vi "加载compactRIOconfig.vi"(8 "error in (no error)":errorcluster caption="错误输入（无错误）") -> (0 "error out":errorcluster caption="错误输出")   [LabVIEW 2014]
doc: "该模板用于创建子VI。"
uses:
  glb/glb_static.vi
  <vilib>/Utility/config.llb/NI_LVConfig.lvlib
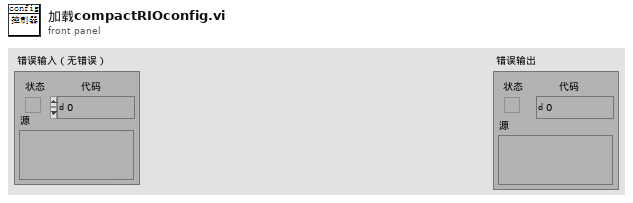
[diagram p1: front panel]
types:
  T1 = typedef "NI_LVConfig.lvlib/Config Data RefNum.ctl" = refnum<k1>
  T2 = cluster{"板卡类型":string, "信号类型":string, "上限":string, "下限":string, "单位":string, "通道数":u32, "最大采样率":u32, "设置采样率":u32, "附加条件":string[], "板卡型号":string}
  T3 = cluster{"控制型号":string, "插槽数目":u32, "板卡信息":cluster{"板卡类型":string, "信号类型":string, "上限":string, "下限":string, "单位":string, "通道数":u32, "最大采样率":u32, "设置采样率":u32, "附加条件":string[], "板卡型号":string}[]}
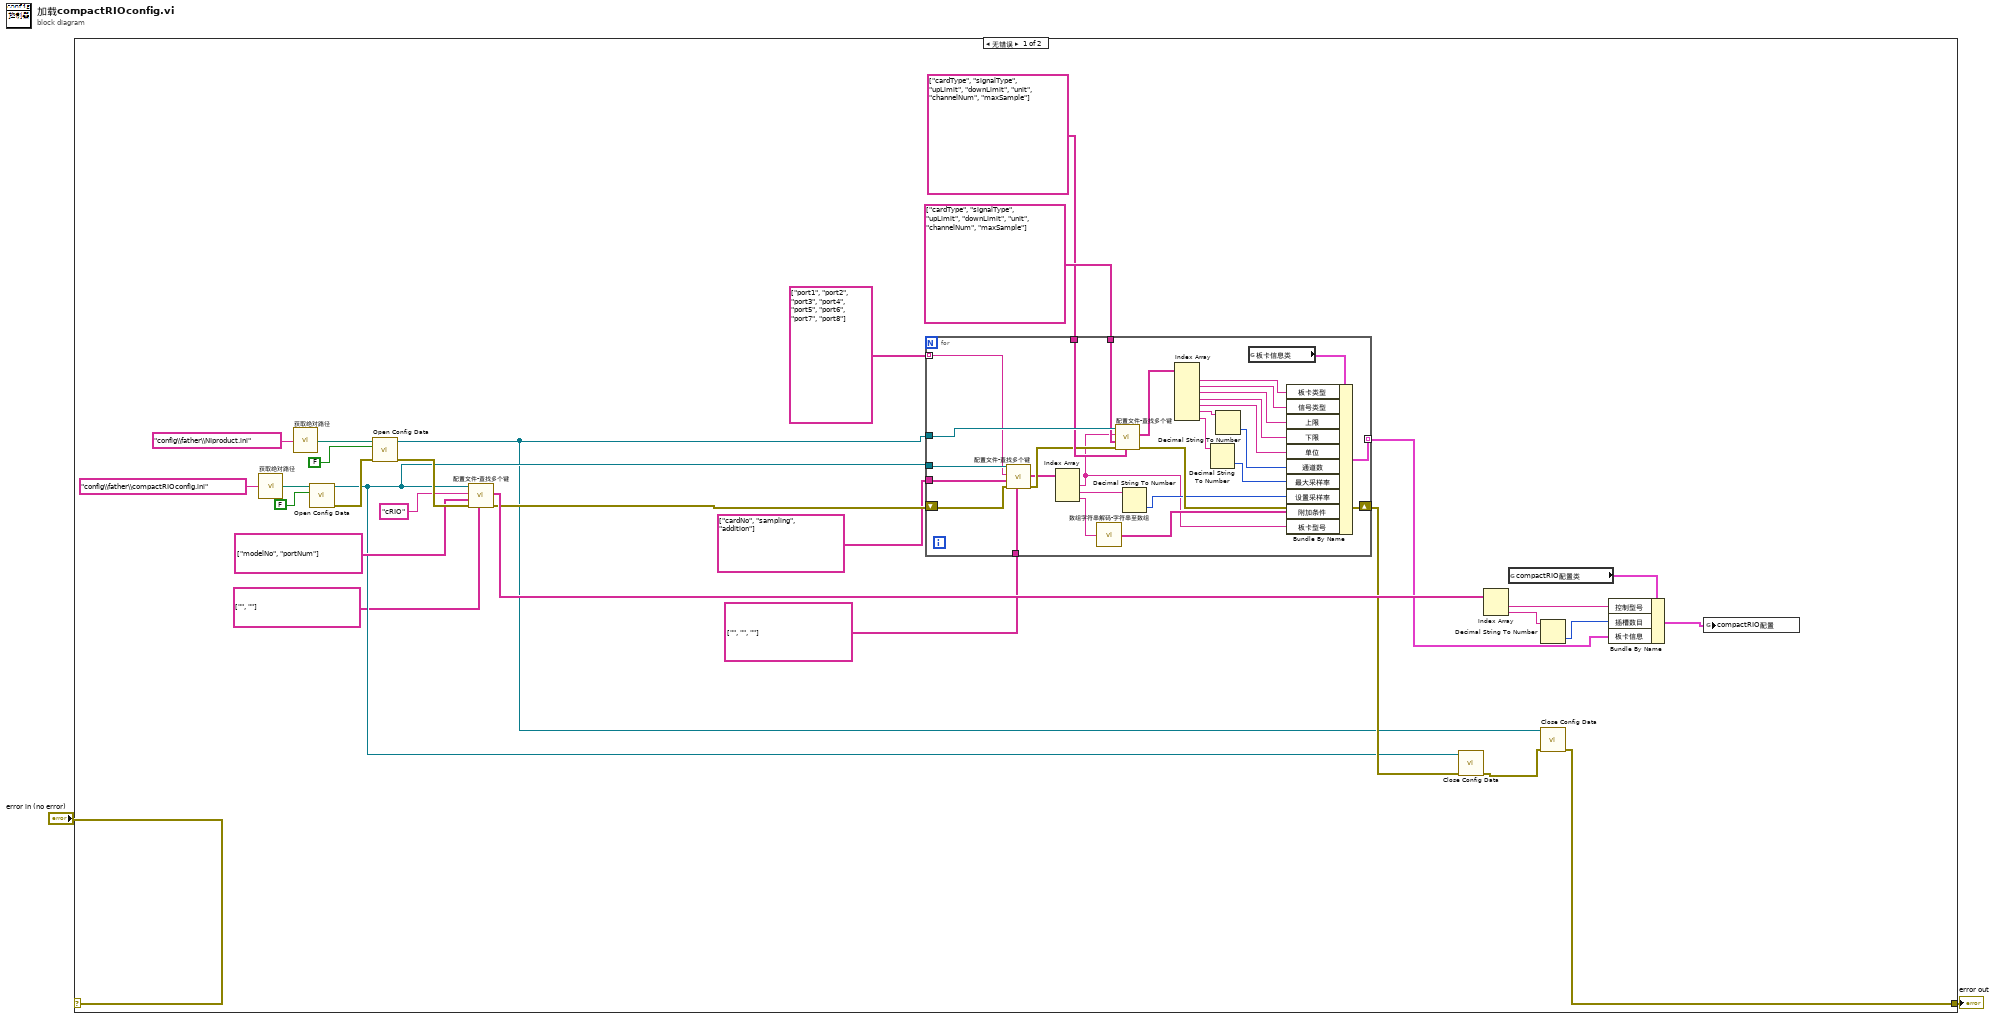
[diagram p0: block diagram]
diagram:
  n1 = case shown="无错误" "error in (no error)" {
    selector: "error in (no error)" -> [_ w60]
    tunnel: [w8 w60] -> w1
    frame No Error {
      n2 = call "获取绝对路径.vi"("relativePath"="config\\father\\compactRIOconfig.ini" ("测试模块配置文件")) -> ("absolutePath"=w31:path)
      n3 = call "获取绝对路径.vi"("relativePath"="config\\father\\NIproduct.ini" ("测试模块配置文件")) -> ("absolutePath"=w26:path)
      n4 = call <vilib>:"Open Config Data.vi"("create file if necessary (T)"=FALSE, "configuration file path"=w31) -> ("error out"=w25:errorcluster, "refnum"=w11:T1)  [unwired: 7 in, 1 out]
      n5 = call <vilib>:"Open Config Data.vi"("error in (no error)"=w25, "create file if necessary (T)"=FALSE, "configuration file path"=w26) -> ("error out"=w24:errorcluster, "refnum"=w9:T1)  [unwired: 6 in, 1 out]
      n6 = call "配置文件-查找多个键.vi"("默认值"=string[] ["", ""], "错误输入（无错误）"=w24, "键名"=string[] ["modelNo", "portNum"], "章名"="cRIO", "引用句柄输入"=w11) -> ("错误输出"=w16:errorcluster, "查询结果"=w21:string[])  [unwired: 4 in, 1 out]
      n7 = for {
        shift-right: [w57] -> w12
        shift-left: w16 -> [w40]
        tunnel: w11 -> [w43]
        tunnel: w9 -> [w59]
        tunnel: string[] ["port1", "port2", "port3", "port4", "port5", "port6", "port7", "port8"] -> [w42] mode=indexing
        tunnel: string[] ["cardType", "signalType", "upLimit", "downLimit", "unit", "channelNum", "maxSample"] -> [w58]
        tunnel: [w45] -> w13 mode=indexing
        tunnel: string[] ["cardType", "signalType", "upLimit", "downLimit", "unit", "channelNum", "maxSample"] -> [w44]
        tunnel: string[] ["cardNo", "sampling", "addition"] -> [w41]
        tunnel: string[] ["", "", ""] -> [w39]
        n8 = call "配置文件-查找多个键.vi"("默认值"=w39, "错误输入（无错误）"=w40, "键名"=w41, "章名"=w42, "引用句柄输入"=w43) -> ("错误输出"=w38:errorcluster, "查询结果"=w37:string[])  [unwired: 4 in, 1 out]
        n9 = Index Array(array=w37) -> (element #1=w32:string, element #2=w35:string, element #3=w36:string)  [unwired: 3 in]
        n10 = call "数组字符串解码-字符串至数组.vi"("字符串"=w36) -> ("数组"=w33:string[])  [unwired: 1 in]
        n11 = call "配置文件-查找多个键.vi"("默认值"=w44, "错误输入（无错误）"=w38, "键名"=w58, "章名"=w32, "引用句柄输入"=w59) -> ("错误输出"=w57:errorcluster, "查询结果"=w55:string[])  [unwired: 4 in, 1 out]
        n12 = Decimal String To Number(string=w35) -> (number=w34:i32)  [unwired: 2 in, 1 out]
        n13 = Index Array(array=w55) -> (element #1=w54:string, element #2=w53:string, element #3=w52:string, element #4=w51:string, element #5=w50:string, element #6=w49:string, element #7=w47:string)  [unwired: 7 in]
        n14 = Decimal String To Number(string=w47) -> (number=w46:i32)  [unwired: 2 in, 1 out]
        n15 = Decimal String To Number(string=w49) -> (number=w48:i32)  [unwired: 2 in, 1 out]
        n16 = global read "类信息.vi" "板卡信息类"() -> (w56:T2)
        n17 = Bundle By Name(cluster=w56, "板卡类型"=w54, "信号类型"=w53, "上限"=w52, "下限"=w51, "单位"=w50, "通道数"=w48, "最大采样率"=w46, "设置采样率"=w34, "附加条件"=w33, "板卡型号"=w32) -> (w45:T2)
      }
      n18 = call <vilib>:"Close Config Data.vi"("error in (no error)"=w12, "refnum"=w11) -> ("error out"=w10:errorcluster)  [unwired: 8 in, 1 out]
      n19 = Index Array(array=w21) -> (element #1=w19:string, element #2=w18:string)  [unwired: 2 in]
      n20 = global read "类信息.vi" "compactRIO配置类"() -> (w20:T3)
      n21 = Decimal String To Number(string=w18) -> (number=w17:i32)  [unwired: 2 in, 1 out]
      n22 = call <vilib>:"Close Config Data.vi"("error in (no error)"=w10, "refnum"=w9) -> ("error out"=w8:errorcluster)  [unwired: 8 in, 1 out]
      n23 = Bundle By Name(cluster=w20, "控制型号"=w19, "插槽数目"=w17, "板卡信息"=w13) -> (w7:T3)
      n24 = global write "glb_static.vi" "compactRIO配置"(w7) -> ()
    }
    frame Error {
    }
  }
  "error out" <- w1
